vi "queue sm 6.vi"() -> ()   [LabVIEW 2020]
uses:
  file I O/ASSIGN 8/que sm states.ctl
panel:
  out "data state 2":i32[][](array[numeric])
  out "data state 1":i32[][](array[numeric])
  out "data init":i32[][](array[numeric])
  out "State output":string
  out "state":T1
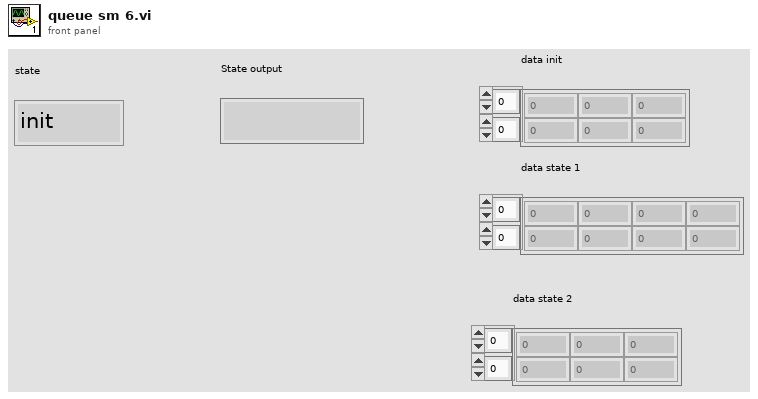
[diagram p1: front panel]
types:
  T1 = typedef "que sm states.ctl" = enum16{"init", "events", "state 1", "state 2", "stop"}
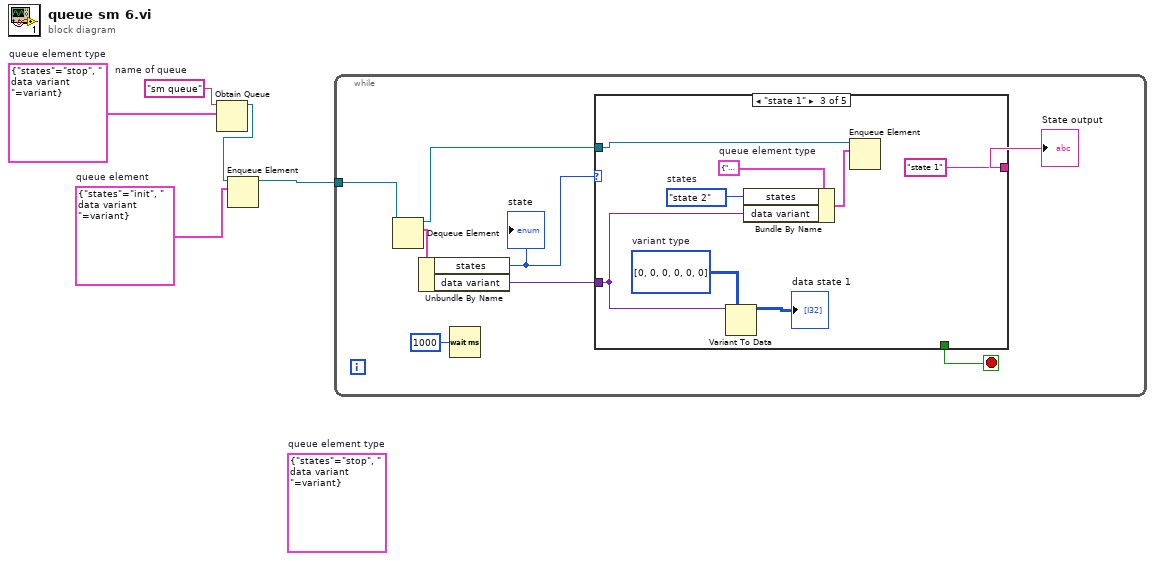
[diagram p0: block diagram]
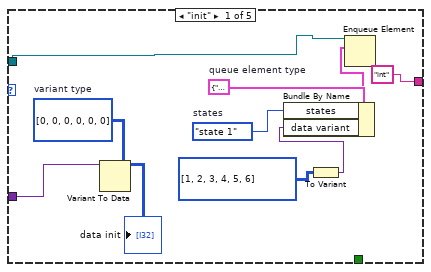
[diagram p2: hidden frame]
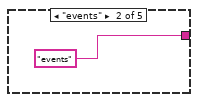
[diagram p3: hidden frame]
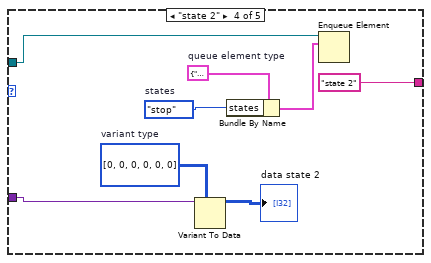
[diagram p4: hidden frame]
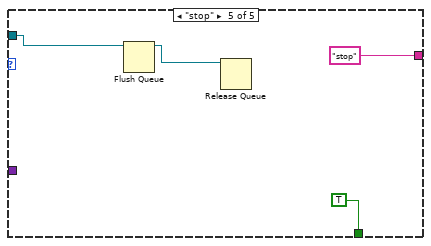
[diagram p5: hidden frame]
diagram:
  (unwired) cluster{"states":T1, " data variant ":variant} {"states"=enum."stop", " data variant "=variant(i32[][] [[0, 0, 0], [0, 0, 0]])}  # queue element type
  w1 = cluster{"states":T1, " data variant ":variant} {"states"=enum."init", " data variant "=variant(i32[][] [[0, 0, 0], [0, 0, 0]])}  # queue element
  w4 = "sm queue"  # name of queue
  w5 = cluster{"states":T1, " data variant ":variant} {"states"=enum."stop", " data variant "=variant(i32[][] [[0, 0, 0], [0, 0, 0]])}  # queue element type
  n1 = Obtain Queue(name (unnamed)=w4, element data type=w5) -> (queue out=w3:refnum<queue>)  [unwired: 3 in, 2 out]
  n2 = Enqueue Element(queue=w3, element=w1) -> (queue out=w2:refnum<queue>)  [unwired: 2 in, 2 out]
  n3 = while {
    tunnel: w2 -> [w10]
    stop <- w7 stop-if-true
    n4 = Dequeue Element(queue=w10) -> (queue out=w9:refnum<queue>, element=w13:cluster{"states":T1, " data variant ":variant})  [unwired: 2 in, 2 out]
    n5 = Unbundle By Name(w13) -> ("states"=w8:T1, "data variant"=w6:variant)
    "state" <- w8
    n6 = Wait (ms)(milliseconds to wait=u32 1000) -> ()  [unwired: 1 out]
    n7 = case shown="\"state 1\"" w8 {
      tunnel: w9 -> [w18 _ w31 w34 w42]
      tunnel: ["int" "events" "state 1" "state 2" "stop"] -> w11
      tunnel: [_ _ _ _ TRUE] -> w7
      tunnel: w6 -> [w20 _ w25 w33 _]
      frame "init" {
        w16 = que_sm_states."state 1"  # states
        w19 = cluster{"states":T1, " data variant ":variant} {"states"=enum."stop", " data variant "=variant(i32[][] [[0, 0, 0], [0, 0, 0]])}  # queue element type
        w22 = i32[][] [[0, 0, 0], [0, 0, 0]]  # variant type
        n8 = Variant To Data(type=w22, Variant=w20) -> (data=→"data init":i32[][])  [unwired: 1 in, 1 out]
        n9 = To Variant(anything=i32[][] [[1, 2, 3], [4, 5, 6]]) -> (Variant=w14:variant)
        n10 = Bundle By Name(cluster=w19, "states"=w16, "data variant"=w14) -> (w17:cluster{"states":T1, " data variant ":variant})
        n11 = Enqueue Element(queue=w18, element=w17) -> ()  [unwired: 2 in, 3 out]
      }
      frame "events" {
      }
      frame "state 1" {
        w27 = i32[][] [[0, 0, 0], [0, 0, 0]]  # variant type
        w28 = cluster{"states":T1, " data variant ":variant} {"states"=enum."stop", " data variant "=variant(i32[][] [[0, 0, 0], [0, 0, 0]])}  # queue element type
        w30 = que_sm_states."state 2"  # states
        n12 = Variant To Data(type=w27, Variant=w25) -> (data=→"data state 1":i32[][])  [unwired: 1 in, 1 out]
        n13 = Bundle By Name(cluster=w28, "states"=w30, "data variant"=w25) -> (w29:cluster{"states":T1, " data variant ":variant})
        n14 = Enqueue Element(queue=w31, element=w29) -> ()  [unwired: 2 in, 3 out]
      }
      frame "state 2" {
        w36 = i32[][] [[0, 0, 0], [0, 0, 0]]  # variant type
        w37 = cluster{"states":T1, " data variant ":variant} {"states"=enum."stop", " data variant "=variant(i32[][] [[0, 0, 0], [0, 0, 0]])}  # queue element type
        w39 = que_sm_states."stop"  # states
        n15 = Variant To Data(type=w36, Variant=w33) -> (data=→"data state 2":i32[][])  [unwired: 1 in, 1 out]
        n16 = Bundle By Name(cluster=w37, "states"=w39) -> (w38:cluster{"states":T1, " data variant ":variant})
        n17 = Enqueue Element(queue=w34, element=w38) -> ()  [unwired: 2 in, 3 out]
      }
      frame "stop" {
        n18 = Flush Queue(queue=w42) -> (queue out=w41:refnum<queue>)  [unwired: 1 in, 2 out]
        n19 = Release Queue(queue=w41) -> ()  [unwired: 2 in, 3 out]
      }
    }
    "State output" <- w11
  }
